vi "member_register.vi"() -> (0 "Cancel":bool, 1 "Username out":string, 2 "Password check pass":bool, 3 "Password empty":bool, 4 "Password out":string, 5 "Username empty":bool)   [LabVIEW 2014]
panel:
  in  "Cancel Button":bool
  in  "OK Button":bool
  in  "Password Check":string
  in  "Your Password":string
  in  "Your Username":string
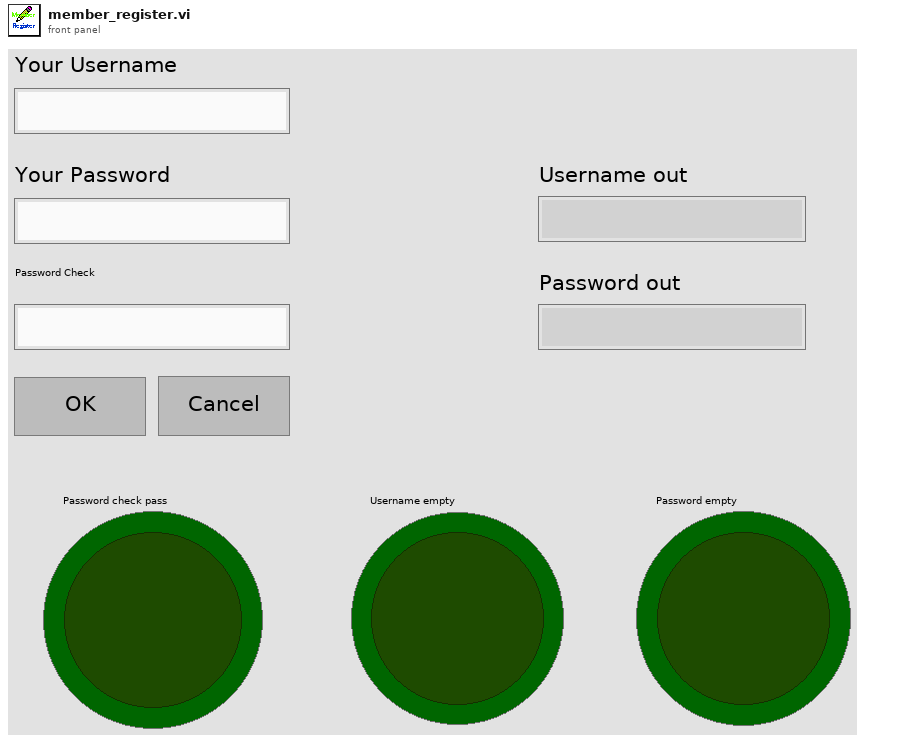
[diagram p1: front panel]
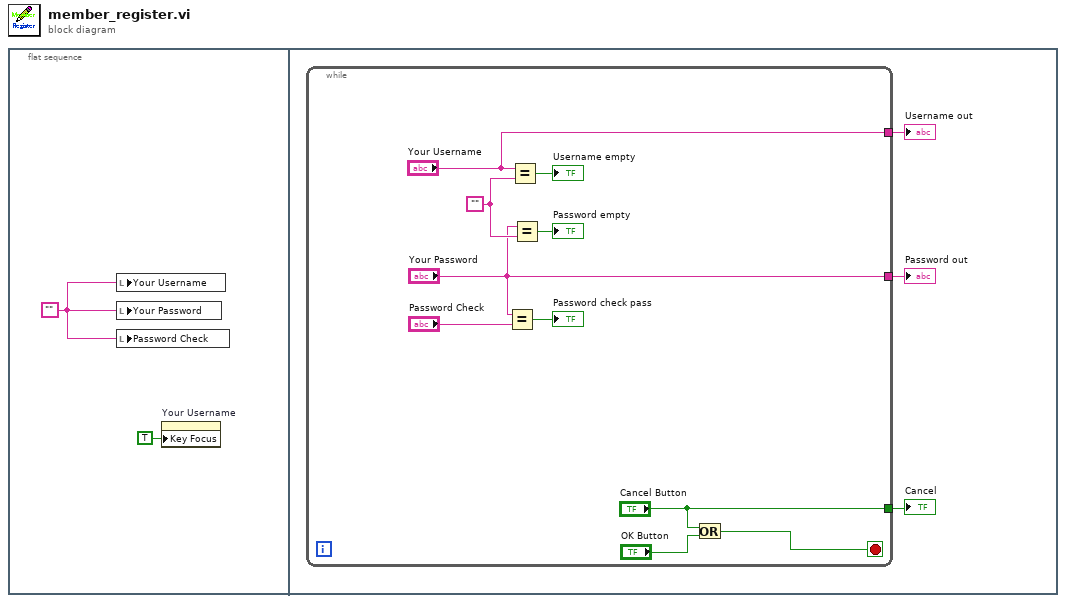
[diagram p0: block diagram]
diagram:
  n1 = flat-sequence {
    frame #0 {
      w2 = ""
      n2 = local write "Your Username"(w2) -> ()
      n3 = local write "Your Password"(w2) -> ()
      n4 = local write "Password Check"(w2) -> ()
      n5 = property on="Your Username" class="Str"("Key Focus"=TRUE) -> ()  [unwired: 2 in, 2 out]
    }
    frame #1 {
      n6 = while {
        tunnel: ["Your Password"] -> w4
        tunnel: ["Your Username"] -> w5
        tunnel: ["Cancel Button"] -> w3
        stop <- w8 stop-if-true
        w13 = ""
        n7 = Equal?(x="Your Password", y="Password Check") -> (x = y?=→"Password check pass":bool)
        n8 = Equal?(x="Your Username", y=w13) -> (x = y?=→"Username empty":bool)
        n9 = Equal?(x="Your Password", y=w13) -> (x = y?=→"Password empty":bool)
        n10 = Or(x="Cancel Button", y="OK Button") -> (x .or. y?=w8:bool)
      }
      "Username out" <- w5
      "Password out" <- w4
      "Cancel" <- w3
    }
  }
